vi "GetChannelIndex.vi"(8 "error in (no error)":errorcluster, 10 "sName":string, 11 "NISTFGenPluginsBase in":refnum<class "NISTFGenPluginsBase.lvclass">) -> (0 "error out":errorcluster, 3 "NISTFGenPluginsBase out":refnum<class "NISTFGenPluginsBase.lvclass">)   [LabVIEW 2014, in "FGenPlugins.lvlib" / "NISTFGenPluginsBase.lvclass"]
uses:
  NISTFGenPluginsBase.lvclass
  <vilib>/Utility/error.llb/Error Cluster From Error Code.vi
  <vilib>/ErrorRing/Error Ring.xnode
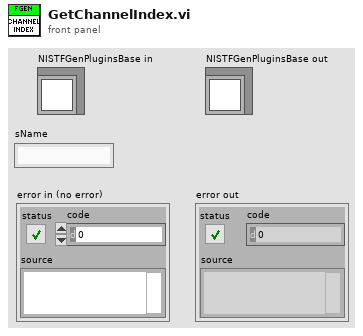
[diagram p1: front panel]
types:
  T1 = typedef "FGenPlugins.lvlib/NISTFGenPluginsBase.lvclass/ChannelParamElement.ctl" = cluster{"sName":string, "eOperateMode":u16, "bEnabled":bool, "eOutputMode":u16, "iIndex":i32, "iNameBufferSize":i32, "fGain":dbl}
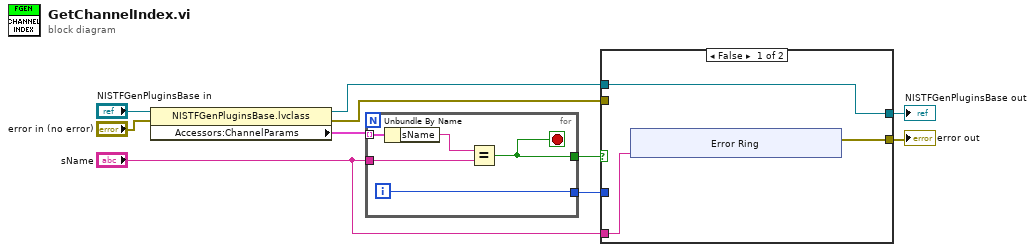
[diagram p0: block diagram]
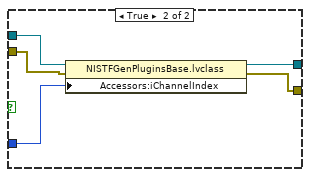
[diagram p2: hidden frame]
diagram:
  n1 = property class="NISTFGenPluginsBase.lvclass"(reference="NISTFGenPluginsBase in", error in="error in (no error)") -> (reference out=w8:refnum<class "NISTFGenPluginsBase.lvclass">, error out=w5:errorcluster, "Accessors:ChannelParams"=w4:T1[])
  n2 = for {
    tunnel: w4 -> [w14] mode=indexing
    tunnel: "sName" -> [w11]
    tunnel: [w15] -> w7
    tunnel: [w12] -> w3
    i -> [w15]
    stop <- w12 stop-if-true
    n3 = Unbundle By Name(w14) -> ("sName"=w13:string)
    n4 = Equal?(x=w13, y=w11) -> (x = y?=w12:bool)
  }
  n5 = case shown="False" w3 {
    tunnel: w8 -> [w18 w30]
    tunnel: w7 -> [_ w29]
    tunnel: [w18 w28] -> w6
    tunnel: w5 -> [_ w27]
    tunnel: "sName" -> [w17 _]
    tunnel: [w16 w26] -> w2
    frame False {
      n6 = xnode "Error Ring"("parameter 0"=w17) -> ("error out"=w16:errorcluster)
    }
    frame True {
      n7 = property class="NISTFGenPluginsBase.lvclass"(reference=w30, error in=w27, "Accessors:iChannelIndex"=w29) -> (reference out=w28:refnum<class "NISTFGenPluginsBase.lvclass">, error out=w26:errorcluster)
    }
  }
  "NISTFGenPluginsBase out" <- w6
  "error out" <- w2
